vi "sig_test.vi"(2 "index (row)":i32) -> (0 "element":dbl format="%#_16f")   [LabVIEW 2010]
panel:
  out "array":dbl[][](array[numeric]) format="%_16f"
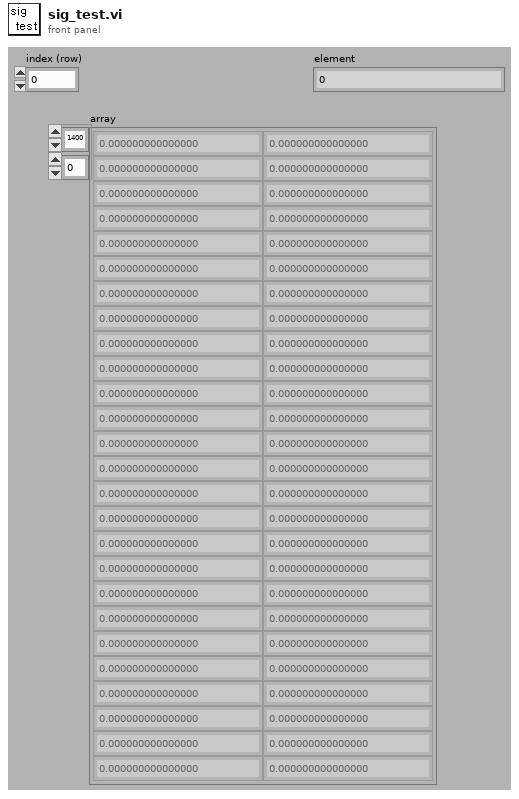
[diagram p1: front panel]
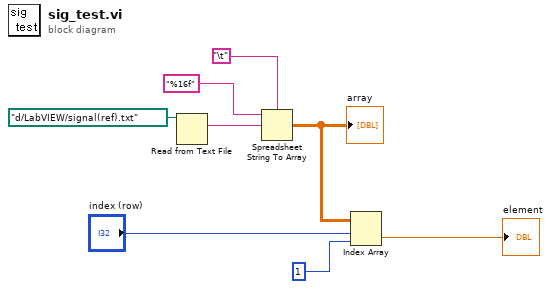
[diagram p0: block diagram]
diagram:
  n1 = Read from Text File(file (use dialog)=path "d:/LabVIEW/signal(ref).txt") -> (text=w7:string)  [unwired: 3 in, 3 out]
  n2 = Spreadsheet String To Array(delimiter (Tab)="\t", format string="%16f", spreadsheet string=w7) -> (array=w4:dbl[][])  [unwired: 1 in]
  "array" <- w4
  n3 = Index Array(array=w4, index (row)="index (row)", index (col)=1 ("disabled index (col)")) -> (element=→"element":dbl)
